vi "fgv_pos_reference.vi"(7 "State":enum16{"Initialise", "Write", "Read", "Clear"}(ring), 8 "error in (no error)":errorcluster, 11 "Pos ref in":sgl[](array[numeric])) -> (0 "error in (no error)":errorcluster, 2 "Pos Value":sgl, 3 "Pos ref out":sgl[][](array[numeric]))   [LabVIEW 2020]
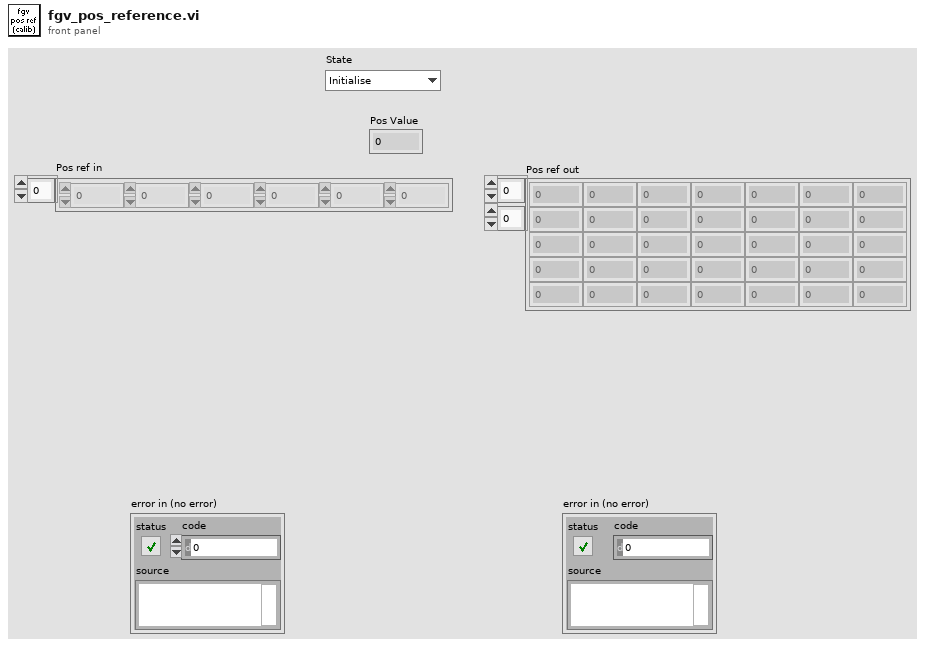
[diagram p1: front panel]
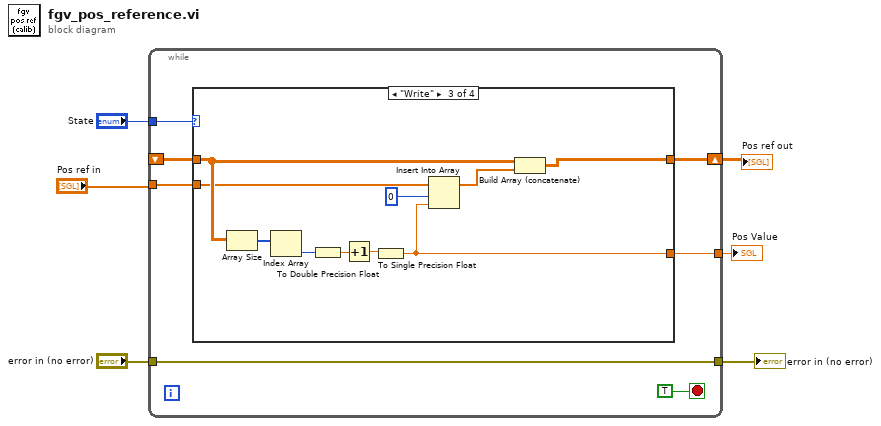
[diagram p0: block diagram]
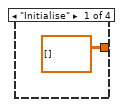
[diagram p2: hidden frame]
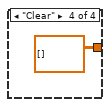
[diagram p4: hidden frame]
diagram:
  n1 = while {
    tunnel: "State" -> [w12]
    tunnel: "Pos ref in" -> [w11]
    shift-right: [w10] -> w5
    shift-left: _ -> [w9]
    tunnel: "error in (no error)" -> [w8]
    tunnel: [w8] -> w3
    tunnel: [w7] -> w1
    stop <- TRUE stop-if-true
    n2 = case shown="\"Write\"" w12 {
      tunnel: w11 -> [_ _ w21 _]
      tunnel: [sgl[][] [] w15 w25 sgl[][] []] -> w10
      tunnel: w9 -> [_ w15 w24 _]
      tunnel: [_ _ w16 _] -> w7
      frame "Initialise" {
      }
      frame "Read", Default {
      }
      frame "Write" {
        n3 = Array Size(array=w24) -> (size(s)=w23:i32[])
        n4 = Index Array(array=w23) -> (element=w22:i32)  [unwired: 1 in]
        n5 = To Double Precision Float(number=w22) -> (double precision float=w19:dbl)
        n6 = Increment(x=w19) -> (x+1=w18:dbl)
        n7 = To Single Precision Float(number=w18) -> (single precision float=w16:sgl)
        n8 = Insert Into Array(array=w21, index=0, new element=w16) -> (w20:sgl[])
        n9 = Build Array (concatenate)(w24, w20) -> (w25:sgl[][])
      }
      frame "Clear" {
      }
    }
  }
  "error in (no error)" <- w3
  "Pos ref out" <- w5
  "Pos Value" <- w1
